vi "Kicker_Release_Kicking_Plate.vi"(8 "error in":errorcluster, 10 "Release Mag":bool=TRUE, 11 "Required Pos":dbl(slide)=20.0 step=0.1 scale=0.0..100.0 scale format="%#_3g%%") -> (0 "error out":errorcluster, 3 "Pot Position":dbl format="%#_3g")   [LabVIEW 2017]
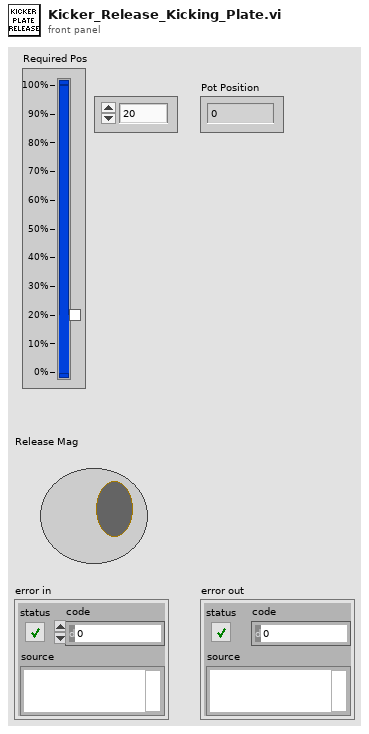
[diagram p1: front panel]
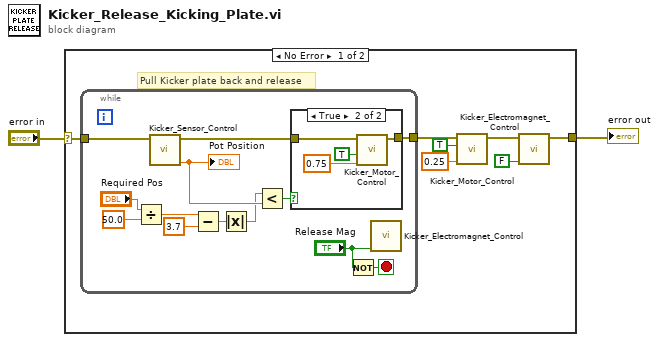
[diagram p0: block diagram]
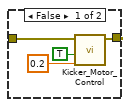
[diagram p2: hidden frame]
diagram:
  n1 = case shown="No Error" "error in" {
    selector: "error in" -> [w3 w31]
    tunnel: [w8 w31] -> w2
    frame No Error {
      # "Pull Kicker plate back and release"
      n2 = while {
        tunnel: [w17] -> w6
        tunnel: w3 -> [w20]
        stop <- w21 stop-if-true
        n3 = Divide(x="Required Pos", y=50.0) -> (x/y=w15:dbl)
        n4 = call "Kicker_Sensor_Control.vi"("error in"=w20) -> ("Pot Output"=w19:dbl, "error out"=w18:errorcluster)  [unwired: 9 in]
        "Pot Position" <- w19
        n5 = Subtract(x=w15, y=3.7) -> (x-y=w14:dbl)
        n6 = Absolute Value(x=w14) -> (abs(x)=w10:dbl)
        n7 = Less?(x=w10, y=w19) -> (x < y?=w22:bool)
        n8 = case shown="True" w22 {
          tunnel: w18 -> [w24 w28]
          tunnel: [w23 w27] -> w17
          frame False {
            n9 = call "Kicker_Motor_Control.vi"("Duty Cycle"=0.2, "Motor Dir"=TRUE, "error in"=w24) -> ("error out"=w23:errorcluster)  [unwired: 8 in]
          }
          frame True {
            n10 = call "Kicker_Motor_Control.vi"("Duty Cycle"=0.75, "Motor Dir"=TRUE, "error in"=w28) -> ("error out"=w27:errorcluster)  [unwired: 8 in]
          }
        }
        n11 = Not(x="Release Mag") -> (.not. x?=w21:bool)
        n12 = call "Kicker_Electromagnet_Control.vi"("Mag Enable"="Release Mag") -> ()  [unwired: 10 in, 1 out]
      }
      n13 = call "Kicker_Motor_Control.vi"("Duty Cycle"=0.25, "Motor Dir"=TRUE, "error in"=w6) -> ("error out"=w7:errorcluster)  [unwired: 8 in]
      n14 = call "Kicker_Electromagnet_Control.vi"("Mag Enable"=FALSE ("A/DIO6 (Pin 23)"), "error in"=w7) -> ("error out"=w8:errorcluster)  [unwired: 9 in]
    }
    frame Error {
    }
  }
  "error out" <- w2
